vi "ELEC_DELAY.vi"(0 "VISA IN":refnum<visa-resource-name>, 1 "Delay(sec)":dbl, 2 "Velocity Factor":dbl, 3 "Media":string(combo), 4 "Cutoff Frq.":dbl, 5 "error in":errorcluster, 7 "Channel":i32=1) -> (14 "VISA Out":refnum<visa-resource-name>, 19 "error out":errorcluster)   [LabVIEW 2018, in "PNA-X.lvlib"]
uses:
  PNA-X.lvlib
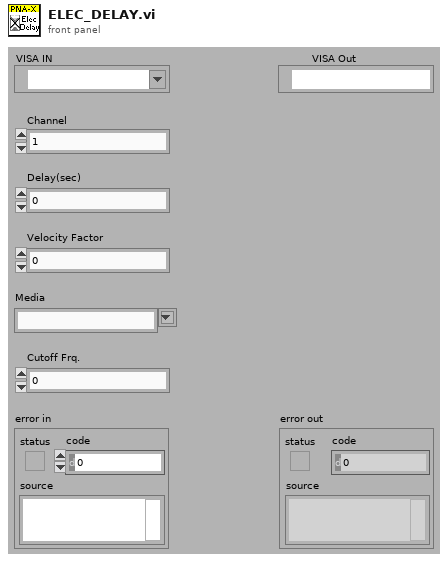
[diagram p1: front panel]
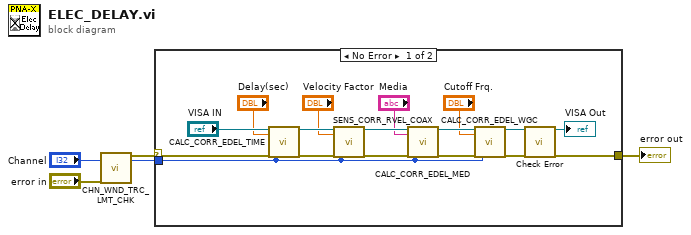
[diagram p0: block diagram]
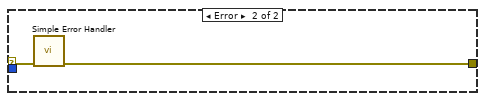
[diagram p2: hidden frame]
diagram:
  n1 = call "CHN_WND_TRC_LMT_CHK.vi"("Channel"="Channel", "error in"="error in") -> ("error out"=w2:errorcluster, "Channel"=w1:i32)  [unwired: 13 in, 3 out]
  n2 = case shown="No Error" w2 {
    selector: w2 -> [w20 w24]
    tunnel: [w22 w23] -> w4
    tunnel: w1 -> [w10 _]
    frame No Error {
      n3 = call "CALC_CORR_EDEL_TIME.vi"("VISA IN"="VISA IN", "Delay(sec)"="Delay(sec)", "error in"=w20, "Channel"=w10) -> ("VISA Out"=w14:refnum<visa-resource-name>, "error out"=w19:errorcluster)  [unwired: 14 in]
      n4 = call "SENS_CORR_RVEL_COAX.vi"("VISA IN"=w14, "Velocity Factor"="Velocity Factor", "error in"=w19, "Channel"=w10) -> ("VISA Out"=w13:refnum<visa-resource-name>, "error out"=w18:errorcluster)  [unwired: 14 in]
      n5 = call "CALC_CORR_EDEL_MED.vi"("VISA IN"=w13, "Media"="Media", "error in"=w18, "Channel"=w10) -> ("VISA Out"=w12:refnum<visa-resource-name>, "error out"=w17:errorcluster)  [unwired: 14 in]
      n6 = call "CALC_CORR_EDEL_WGC.vi"("VISA IN"=w12, "Cutoff Frq."="Cutoff Frq.", "error in"=w17, "Channel"=w10) -> ("VISA Out"=w11:refnum<visa-resource-name>, "error out"=w16:errorcluster)  [unwired: 14 in]
      n7 = call "Check Error.vi"("VISA Resource Name"=w11, "error in (no error)"=w16) -> ("dup VISA session"=→"VISA Out":refnum<visa-resource-name>, "error out"=w22:errorcluster)  [unwired: 16 in]
    }
    frame Error {
      n8 = call <vilib>:"Simple Error Handler.vi"("error in (no error)"=w24) -> ("error out"=w23:errorcluster)  [unwired: 4 in, 4 out]
    }
  }
  "error out" <- w4
